vi "GenerateData.vi"() -> ()   [LabVIEW 2013]
panel:
  out "Booléen":bool
  out "Données":dbl
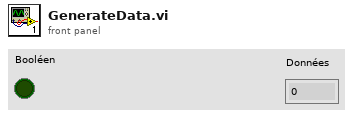
[diagram p1: front panel]
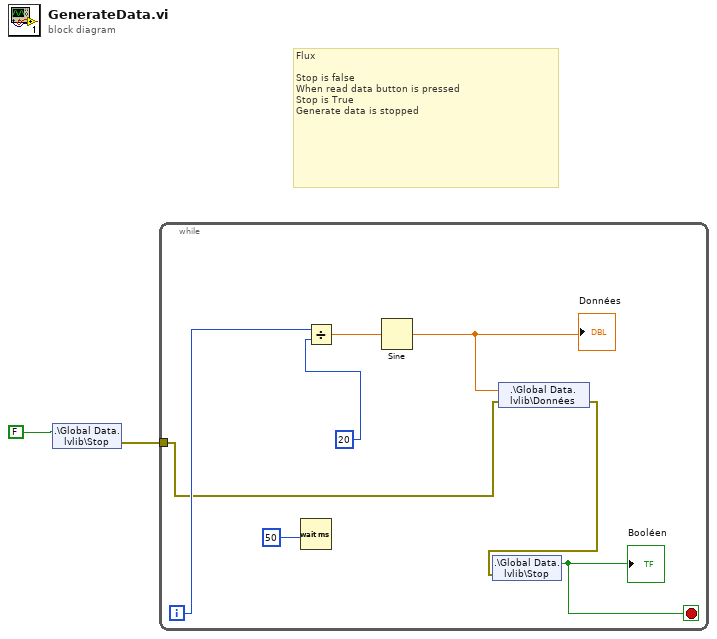
[diagram p0: block diagram]
diagram:
  # "Flux\n\nStop is false\nWhen read data button is pressed\nStop is True\nGenerate data is stopped"
  n1 = shared-variable ".\\Global Data.lvlib\\Stop"(FALSE) -> (error out=w1:errorcluster)  [unwired: 1 in]
  n2 = while {
    tunnel: w1 -> [w5]
    i -> [w9]
    stop <- w3 stop-if-true
    n3 = Wait (ms)(milliseconds to wait=50) -> ()  [unwired: 1 out]
    n4 = Divide(x=w9, y=20) -> (x/y=w7:dbl)
    n5 = Sine(x=w7) -> (sin(x)=w6:dbl)
    "Données" <- w6
    n6 = shared-variable ".\\Global Data.lvlib\\Données"(w6, error in=w5) -> (error out=w4:errorcluster)
    n7 = shared-variable ".\\Global Data.lvlib\\Stop"(error in=w4) -> (w3:bool)  [unwired: 1 out]
    "Booléen" <- w3
  }
